vi "0-Draw Waypoints.vi"(4 "Image Descriptor":T3={"Upper-Left Corner Coordinates"={"UTM Zone"=0.0, "Hemisphere"=enum."North", "East"=0.0, "North"=0.0}, "Meters/Pixel"=42.294203} {"Upper-Left Corner Coordinates"."North" format="%#_10f"; "Upper-Left Corner Coordinates"."East" format="%#_8f"}, 5 "Waypoints List":T2, 6 "Current Waypoint #":T1=-1, 7 "Image In":T5) -> (1 "Coordinate Outside Image":bool, 3 "Image Out":T5)   [LabVIEW 2011]
doc: "Overlays waypoints onto the map image."
uses:
  <vilib>/vision/Image Controls.llb/IMAQ Image.ctl
  0-Image Descriptor.ctl
  2-Think/2 Typedefs/UTM Location.ctl
  0x2-OCU-Think Comm/0x2 Typedefs/Waypoints List.ctl
  2-Think/2 Classes/Waypoint/Waypoint.lvclass
  0x2-OCU-Think Comm/0x2 Typedefs/Current Waypoint.ctl
  2-Think/2 Globals/2 Global.vi
panel:
  in  "Shifted Waypt Color":u32(colorbox)=16776704
  in  "Current Waypt Color":u32(colorbox)=1985280
  in  "Finished Waypt Color":u32(colorbox)=57855
  in  "Waypt Color":u32(colorbox)=16711680
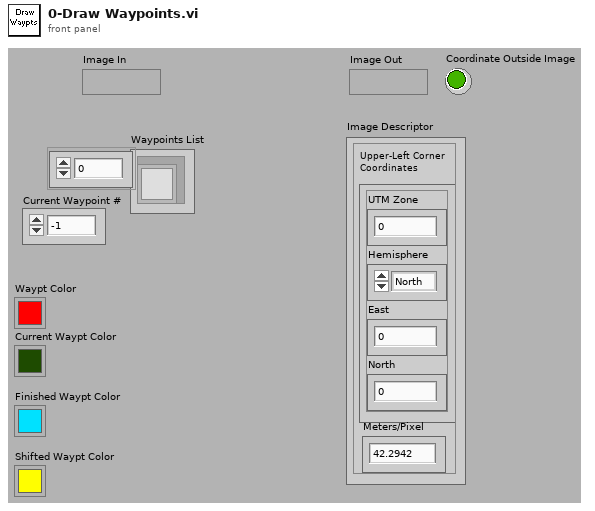
[diagram p1: front panel]
types:
  T1 = typedef "Current Waypoint.ctl" = i32
  T2 = typedef "Waypoints List.ctl" = refnum<class "Waypoint.lvclass">[]
  T3 = typedef "0-Image Descriptor.ctl" = cluster{"Upper-Left Corner Coordinates":T4, "Meters/Pixel":dbl}
  T4 = typedef "UTM Location.ctl" = cluster{"UTM Zone":dbl, "Hemisphere":enum16{"North", "South"}, "East":dbl, "North":dbl}
  T5 = typedef "IMAQ Image.ctl" = refnum<image>
  T6 = cluster{"Desired Font (Application)":enum16{"User-specified Font", "Application Font", "System Font", "Dialog Font"}, "[User-specified Font]":cluster{"Font Name":string, "Size":i16, "Strikeout?":bool, "Italic?":bool, "Underline?":bool, "Outline?":bool, "Shadow?":bool, "Bold?":bool, "Rotation Angle":dbl}, "Horizontal Alignment":i16, "Vertical Alignment":i16}
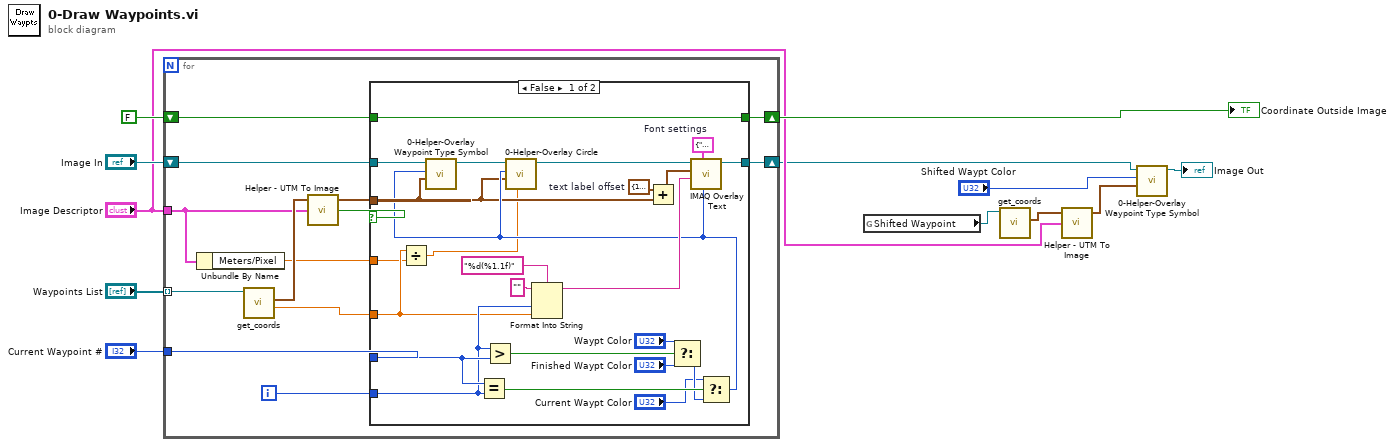
[diagram p0: block diagram]
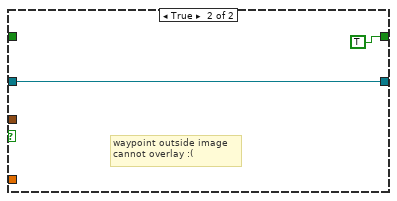
[diagram p2: hidden frame]
diagram:
  n1 = for {
    tunnel: "Waypoints List" -> [w15] mode=indexing
    shift-right: [w24] -> w2
    shift-left: "Image In" -> [w25]
    tunnel: "Image Descriptor" -> [w14]
    tunnel: "Current Waypoint #" -> [w23]
    shift-right: [w20] -> w9
    shift-left: FALSE -> [w19]
    i -> [w18]
    n2 = Unbundle By Name(w14) -> ("Meters/Pixel"=w13:dbl)
    n3 = call-dynamic "get_coords.vi"("Waypoint in"=w15) -> ("Tolerance (meters?)"=w16:dbl, "Coords"=w17:T4)  [unwired: 7 in, 2 out]
    n4 = call "Helper - UTM To Image.vi"("Image Descriptor"=w14, "UTM Location"=w17) -> ("Coordinate Outside Image"=w21:bool, "Pixel Coordinates"=w22:cluster{"X":i32, "Y":i32})  [unwired: 1 in, 1 out]
    n5 = case shown="False" w21 {
      tunnel: w25 -> [w35 w51]
      tunnel: [w46 w51] -> w24
      tunnel: w16 -> [w28 _]
      tunnel: w23 -> [w41 _]
      tunnel: w22 -> [w29 _]
      tunnel: [w36 TRUE] -> w20
      tunnel: w19 -> [w36 _]
      tunnel: w18 -> [w33 _]
      tunnel: w13 -> [w27 _]
      frame False {
        w49 = T6 {"Desired Font (Application)"=enum."User-specified Font", "[User-specified Font]"={"Font Name"="Arial Unicode MS", "Size"=40, "Strikeout?"=FALSE, "Italic?"=FALSE, "Underline?"=FALSE, "Outline?"=FALSE, "Shadow?"=FALSE, "Bold?"=TRUE, "Rotation Angle"=0.0}, "Horizontal Alignment"=0, "Vertical Alignment"=0}  # Font settings
        w48 = cluster{"X":i32, "Y":i32} {"X"=10, "Y"=21}  # text label offset
        n6 = Divide(x=w28, y=w27) -> (x/y=w26:dbl)
        n7 = Equal?(x=w41, y=w33) -> (x = y?=w40:bool)
        n8 = Greater?(x=w33, y=w41) -> (0:w44:bool)
        n9 = Format Into String(format string="%d(%1.1f)", initial string="", w33, w28) -> (resulting string=w37:string)  [unwired: 1 in, 1 out]
        n10 = Add(x=w48, y=w29) -> (x+y=w47:cluster{"X":i32, "Y":i32})
        n11 = Select(t="Waypt Color", s=w44, f="Finished Waypt Color") -> (s? t:f=w39:u32)
        n12 = Select(t="Current Waypt Color", s=w40, f=w39) -> (s? t:f=w30:u32)
        n13 = call "0-Helper-Overlay Waypoint Type Symbol.vi"("Overlay Location"=w29, "Icon Color"=w30, "Image in"=w35) -> ("Image out"=w32:T5)  [unwired: 7 in, 1 out]
        n14 = call "0-Helper-Overlay Circle.vi"("Radius (px)"=w26, "Pixel Coordinates"=w29, "Color"=w30, "Image in"=w32) -> ("Image out"=w31:T5)  [unwired: 7 in]
        n15 = call "IMAQ Overlay Text"("Text Color (black)"=w30, "Font, Size & Style"=w49, "String"=w37, "Origin"=w47, "Image"=w31) -> ("Image Out"=w46:T5)  [unwired: 3 in, 3 out]
      }
      frame True {
        # "waypoint outside image\ncannot overlay :("
      }
    }
  }
  "Coordinate Outside Image" <- w9
  n16 = global read "2 Global.vi" "Shifted Waypoint"() -> (w6:refnum<class "Waypoint.lvclass">)
  n17 = call-dynamic "get_coords.vi"("Waypoint in"=w6) -> ("Coords"=w5:T4)  [unwired: 7 in, 3 out]
  n18 = call "Helper - UTM To Image.vi"("Image Descriptor"="Image Descriptor", "UTM Location"=w5) -> ("Pixel Coordinates"=w3:cluster{"X":i32, "Y":i32})  [unwired: 1 in, 2 out]
  n19 = call "0-Helper-Overlay Waypoint Type Symbol.vi"("Overlay Location"=w3, "Icon Color"="Shifted Waypt Color", "Image in"=w2) -> ("Image out"=→"Image Out":T5)  [unwired: 7 in, 1 out]
